vi "Viewey_Vision.vi"(9 "Smart Dashboard Name":string="VieweyVision", 10 "Settings File":string="VieweyConfig.csv", 11 "Threshold":sgl(knob)=100.0 scale=0.0..200.0) -> ()   [LabVIEW 2016]
uses:
  <vilib>/vision/driver/NI_Vision_Acquisition_Software.lvlib
  <vilib>/vision/driver/IMAQdx.llb/IMAQdx Camera Control Mode.ctl
  <vilib>/userdefined/High Color/IMAQdx.ctl
  <vilib>/vision/NI_Vision_Development_Module.lvlib
  <vilib>/Utility/file.llb/Read From Spreadsheet File (string).vi
panel:
  out "Results":cluster{"Triggered":bool, "Score":sgl}[](array[cluster])
  in  "Save Settings On Exit":bool
  in  "stop":bool
  in  "Region Control":u16(ring) items=["Safe Mode", "Control", "Left", "Right"]
  out "FPS":dbl format="%#_3g"
  out "Image":T1(plugin-control)
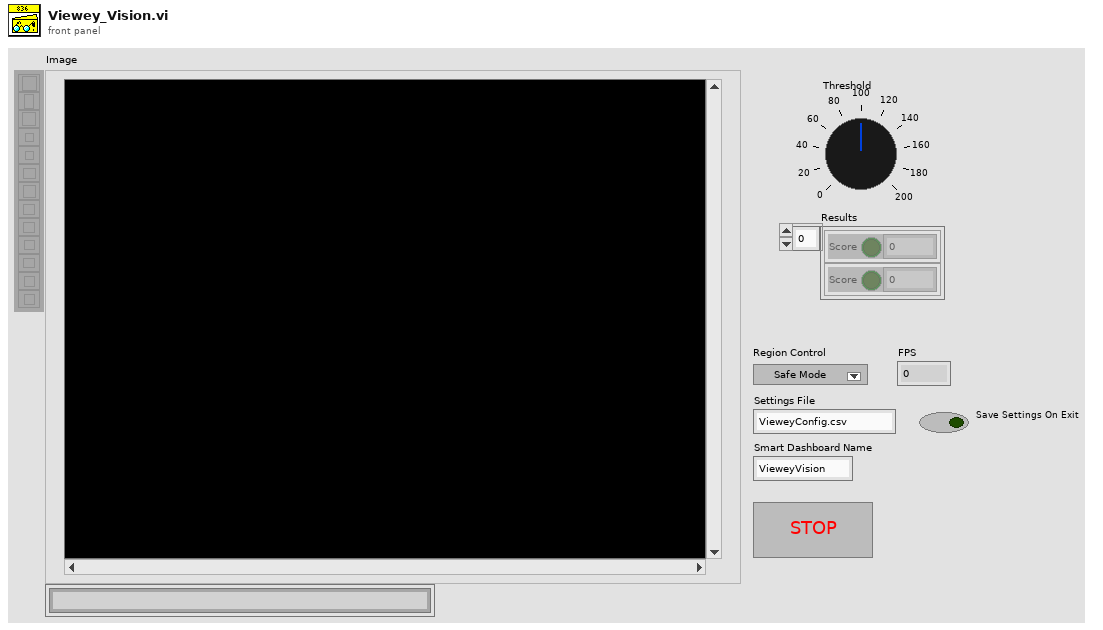
[diagram p1: front panel]
types:
  T1 = typedef "IMAQ Image.ctl" = refnum<image>
  T2 = cluster{"Rectangle Color":u32, "Text Color":u32, "Fill Color":u32}
  T3 = typedef "ROI Descriptor" = cluster{"Global Rectangle":i32[], "Contours":cluster{"ID":enum32{"External", "Internal"}, "Type":u32, "Coordinates":i32[]}[]}
  T4 = typedef "Image Type" = u32
  T5 = typedef "IMAQdx.ctl" = refnum<k21>
  T6 = typedef "NI_Vision_Acquisition_Software.lvlib/IMAQdx Camera Control Mode.ctl" = enum32{"Controller", "Listener"}
  T7 = enum16{"open", "replace", "create", "open or create", "replace or create", "replace or create with confirmation"}
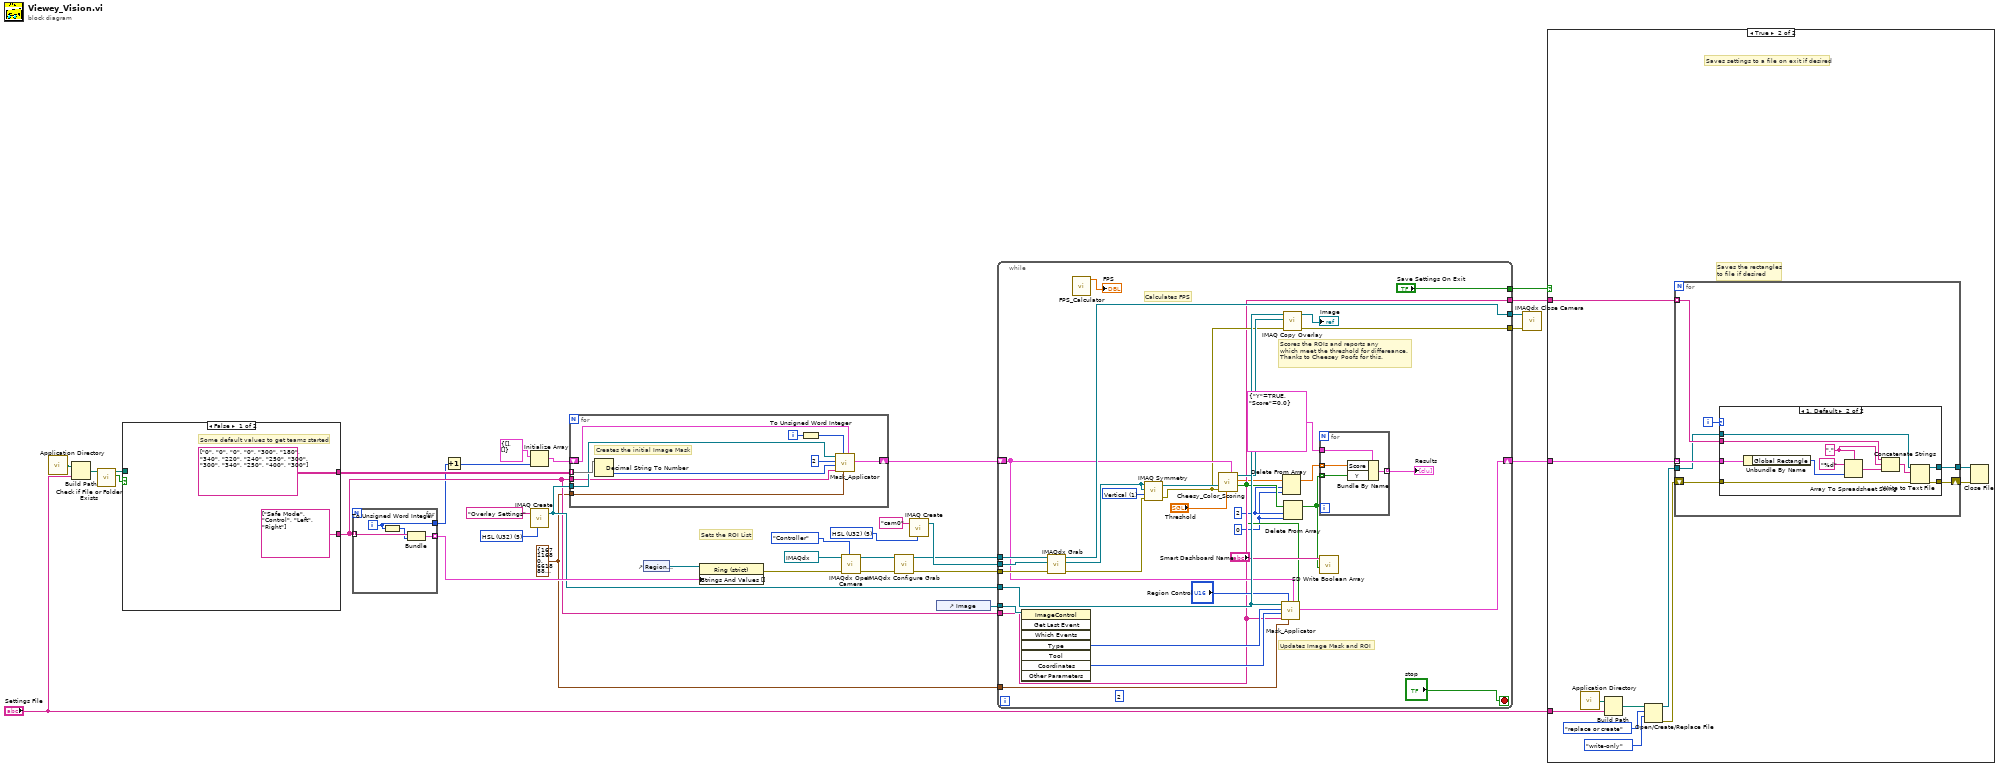
[diagram p0: block diagram]
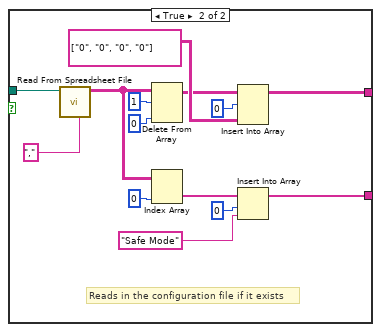
[diagram p2: hidden frame]
diagram:
  w2 = T2 {"Rectangle Color"=16711680, "Text Color"=6618880, "Fill Color"=16776960} ("Cluster")
  w23 = T4 5 items=["Grayscale (U8)", "Grayscale (I16)", "Grayscale (SGL)", "Complex (CSG)", "RGB (U32)", "HSL (U32)", "RGB (U64)", "Grayscale (U16)"] ("Image Type")
  w30 = T4 5 items=["Grayscale (U8)", "Grayscale (I16)", "Grayscale (SGL)", "Complex (CSG)", "RGB (U32)", "HSL (U32)", "RGB (U64)", "Grayscale (U16)"] ("Image Type")
  # "Sets the ROI List"
  n1 = call <vilib>:"Application Directory.vi"() -> ("Application Directory"=w14:path)
  n2 = Build Path(base path=w14, name or relative path="Settings File") -> (appended path=w13:path)
  n3 = call <vilib>:"Check if File or Folder Exists.vi"("path"=w13) -> ("file or folder exists?"=w11:bool, "dup path"=w12:path)  [unwired: 8 in, 1 out]
  n4 = case shown="False" w11 {
    tunnel: w12 -> [_ w50]
    tunnel: [string[] ["Safe Mode", "Control", "Left", "Right"] w46] -> w7
    tunnel: [string[][] [["0", "0", "0", "0"], ["300", "180", "340", "220"], ["240", "250", "300", "300"], ["340", "250", "400", "300"]] ("all rows") w41] -> w10
    frame False {
      # "Some default values to get teams started"
    }
    frame True {
      # "Reads in the configuration file if it exists"
      n5 = call-poly <vilib>:"Read From Spreadsheet File.vi"("delimiter (\\t)"="," ("delimiter (\\t)"), "file path (dialog if empty)"=w50) -> ("all rows"=w40:string[][])  [unwired: 5 in, 4 out]
      n6 = Delete From Array(array=w40, length=1, index (col)=0 ("disabled index (col)")) -> (array with subset deleted=w37:string[][])  [unwired: 1 in, 1 out]
      n7 = Index Array(array=w40, index (col)=0 ("disabled index (col)")) -> (element=w47:string[])  [unwired: 1 in]
      n8 = Insert Into Array(array=w37, index (row)=0, new element=string[][] [["0", "0", "0", "0"]] ("all rows")) -> (w41:string[][])  [unwired: 1 in]
      n9 = Insert Into Array(array=w47, index=0, new element="Safe Mode" ("new element/subarray")) -> (w46:string[])
    }
  }
  n10 = for {
    tunnel: w7 -> [w54] mode=indexing
    tunnel: [w53] -> w20 mode=indexing
    tunnel: [w51] -> w3
    i -> [w51]
    n11 = To Unsigned Word Integer(number=w51) -> (unsigned 16bit integer=w52:u16)
    n12 = Bundle("String"=w54, w52) -> (w53:cluster{"String":string, u16})  [unwired: 1 in]
  }
  n13 = Increment(x=w3) -> (x+1=w1:i32)
  n14 = Initialize Array(T3 {"Global Rectangle"=[], "Contours"=[]} ("element"), w1) -> (w4:T3[])
  n15 = call "IMAQ Create"("Image Name"="Overlay Settings", "Image Type"=w23) -> ("New Image"=w8:T1)  [unwired: 2 in, 2 out]
  n16 = for {
    tunnel: w10 -> [w64] mode=indexing
    tunnel: w8 -> [w63]
    shift-right: [w61] -> w9
    shift-left: w4 -> [w60]
    tunnel: w7 -> [w56]
    tunnel: w2 -> [w55]
    i -> [w58]
    # "Creates the initial Image Mask"
    n17 = Decimal String To Number(string=w64) -> (number=w62:i32[])  [unwired: 2 in, 1 out]
    n18 = To Unsigned Word Integer(number=w58) -> (unsigned 16bit integer=w57:u16)
    n19 = call <userlib>:"Mask_Applicator.vi"("ROI In"=w60, "Cluster"=w55, "ROI Number"=w57, "ROI List In"=w56, "Event Coordinates"=w62, "Event Type"=2, "Image Mask"=w63) -> ("ROI Out"=w61:T3[])  [unwired: 3 in, 1 out]
  }
  n20 = control-ref of="Region Control"() -> (w21:refnum<vi>)
  n21 = property on="Property Node" class="Ring (strict)"(reference=w21, "Strings And Values []"=w20) -> (error out=w22:errorcluster)  [unwired: 1 in, 1 out]
  n22 = call <vilib>:"IMAQdx Open Camera.vi"("Camera Control Mode"=IMAQdx_Camera_Control_Mode."Controller", "error in"=w22, "Session In"=T5 "cam0") -> ("error out"=w28:errorcluster, "Session Out"=w18:T5)  [unwired: 7 in]
  n23 = call <vilib>:"IMAQdx Configure Grab.vi"("error in"=w28, "Session In"=w18) -> ("error out"=w26:errorcluster, "Session Out"=w27:T5)  [unwired: 8 in]
  n24 = call "IMAQ Create"("Image Name"="cam0", "Image Type"=w30) -> ("New Image"=w32:T1)  [unwired: 2 in, 2 out]
  n25 = control-ref of="Image"() -> (w25:refnum<vi>)
  n26 = while {
    tunnel: w26 -> [w98]
    tunnel: [w81] -> w34
    tunnel: w27 -> [w96]
    tunnel: [w95] -> w33
    tunnel: w32 -> [w94]
    tunnel: w25 -> [w93]
    tunnel: w8 -> [w90]
    tunnel: w7 -> [w75]
    shift-right: [w89] -> w17
    shift-left: w9 -> [w87]
    tunnel: [w75] -> w16
    tunnel: ["Save Settings On Exit"] -> w15
    tunnel: w2 -> [w74]
    stop <- "stop" stop-if-true
    (unwired) 2 ("length")
    w66 = 2 ("length")
    w65 = 0 ("index")
    w85 = u32 1 items=["Horizontal", "Vertical", "Central", "1st Diagonal", "2nd Diagonal"] ("Type of Symmetry")
    # "Calculates FPS"
    # "Scores the ROIs and reports any\nwhich meet the threshold for differeance.\nThanks to Cheesey Poofs for this."
    # "Updates Image Mask and ROI"
    n27 = invoke class="ImageControl" method="Get Last Event"(reference=w93) -> ("Type"=w92:i32, "Coordinates"=w86:i32[])  [unwired: 7 in, 6 out]
    n28 = call <vilib>:"IMAQdx Grab.vi"("error in"=w98, "Image In"=w94, "Session In"=w96) -> ("error out"=w82:errorcluster, "Image Out"=w84:T1, "Session Out"=w95:T5)  [unwired: 5 in, 1 out]
    n29 = call <userlib>:"FPS_Calculator.vi"() -> ("FPS"=→"FPS":dbl)  [unwired: 11 in]
    n30 = call "IMAQ Symmetry"("error in (no error)"=w82, "Type of Symmetry"=w85, "Image Dst"=w84, "Image Src"=w84) -> ("error out"=w76:errorcluster, "Image Dst Out"=w80:T1)  [unwired: 1 in]
    n31 = call <userlib>:"Cheesy_Color_Scoring.vi"("ROI Out"=w87, "Threshold"="Threshold", "error in (no error)"=w76, "Source Image In"=w80) -> ("ROI Different"=w71:bool[], "ROI Scores"=w72:sgl[], "Source Image Out"=w77:T1)  [unwired: 5 in]
    n32 = call <userlib>:"Mask_Applicator.vi"("ROI Different"=w71, "ROI In"=w87, "Cluster"=w74, "ROI Number"="Region Control", "ROI List In"=w75, "Event Coordinates"=w86, "Event Type"=w92, "Image Mask"=w90) -> ("ROI Out"=w89:T3[])  [unwired: 2 in, 1 out]
    n33 = Delete From Array(array=w72, length=w66, index=w65) -> (array with subset deleted=w70:sgl[])  [unwired: 1 out]
    n34 = call "IMAQ Copy Overlay"("error in (no error)"=w76, "Image Dst"=w77, "Image Src"=w90) -> ("error out"=w81:errorcluster, "Image Dst Out"=→"Image":T1)  [unwired: 7 in]
    n35 = Delete From Array(array=w71, length=w66, index=w65) -> (array with subset deleted=w69:bool[])  [unwired: 1 out]
    n36 = for {
      tunnel: w70 -> [w101] mode=indexing
      tunnel: w69 -> [w100] mode=indexing
      tunnel: cluster{"Y":bool, "Score":sgl} {"Y"=TRUE, "Score"=0.0} -> [w102]
      tunnel: [w99] -> w67 mode=indexing
      n37 = Bundle By Name(cluster=w102, "Score"=w101, "Y"=w100) -> (w99:cluster{"Y":bool, "Score":sgl})
    }
    "Results" <- w67
    n38 = call <vilib>:"SD Write Boolean Array.vi"("Boolean Array"=w69, "Name"="Smart Dashboard Name") -> ()  [unwired: 8 in, 2 out]
  }
  n39 = call <vilib>:"IMAQdx Close Camera.vi"("error in"=w34, "Session In"=w33) -> ()  [unwired: 9 in, 1 out]
  n40 = case shown="True" w15 {
    tunnel: w17 -> [_ w113]
    tunnel: w16 -> [_ w112]
    tunnel: "Settings File" -> [_ w103]
    frame False {
    }
    frame True {
      # "Saves settings to a file on exit if desired"
      # "Saves the rectangles\nto file if desired"
      n41 = call <vilib>:"Application Directory.vi"() -> ("Application Directory"=w109:path)
      n42 = Build Path(base path=w109, name or relative path=w103) -> (appended path=w108:path)
      n43 = Open/Create/Replace File(file path (use dialog)=w108, operation (0:open)=T7."replace or create", access (0:read/write)=enum16{"read/write", "read-only", "write-only"}."write-only") -> (refnum out=w107:refnum<file>, error out=w106:errorcluster)  [unwired: 3 in, 1 out]
      n44 = for {
        tunnel: w113 -> [w120] mode=indexing
        tunnel: w112 -> [w119] mode=indexing
        tunnel: w107 -> [w118]
        tunnel: [w116] -> w105
        shift-right: [w115] -> w104
        shift-left: w106 -> [w117]
        i -> [w114]
        n45 = case shown="1, Default" w114 {
          tunnel: w120 -> [_ w133]
          tunnel: w119 -> [_ w130]
          tunnel: w118 -> [w122 w128]
          tunnel: w117 -> [w121 w127]
          tunnel: [w122 w126] -> w116
          tunnel: [w121 w125] -> w115
          frame 0 {
          }
          frame 1, Default {
            w123 = "," ("delimiter (Tab)")
            n46 = Unbundle By Name(w133) -> ("Global Rectangle"=w132:i32[])
            n47 = Array To Spreadsheet String(delimiter (Tab)=w123, array=w132, 3:"%d" ("format string")) -> (spreadsheet string=w124:string)
            n48 = Concatenate Strings(w130, w123, w124) -> (w129:string)
            n49 = Write to Text File(file (use dialog)=w128, text=w129, error in=w127) -> (refnum out=w126:refnum<file>, error out=w125:errorcluster)  [unwired: 1 in, 1 out]
          }
        }
      }
      n50 = Close File(refnum=w105, error in=w104) -> ()  [unwired: 2 out]
    }
  }
